vi "Get Stream.vi"(8 "error in (no error)":errorcluster, 11 "Mux in":refnum<class "Mux.lvclass">) -> (0 "error out":errorcluster, 2 "Stream":refnum<class "Stream.lvclass">, 3 "Mux out":refnum<class "Mux.lvclass">)   [LabVIEW 2022 SP3, in "VideoMux.lvlib" / "Mux.lvclass"]
uses:
  Mux.lvclass
  <vilib>/IlluminatedG/lv-stream/stream/Stream.lvclass
  Mux.lvclass/Mux.ctl
  <vilib>/IlluminatedG/lv-stream/Connection/Connection.lvclass
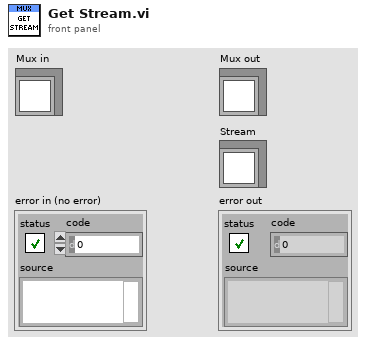
[diagram p1: front panel]
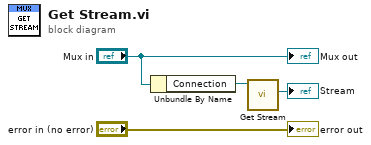
[diagram p0: block diagram]
diagram:
  n1 = Unbundle By Name("Mux in") -> ("Connection"=w2:refnum<class "Connection.lvclass">)
  n2 = call-dynamic "Get Stream.vi"("Connection in"=w2) -> ("Stream"=→"Stream":refnum<class "Stream.lvclass">)  [unwired: 8 in, 2 out]
  "error out" <- "error in (no error)"
  "Mux out" <- "Mux in"
